vi "Get JSON Data.vi"(6 "Force Hide":bool, 7 "Evaluate Pane Move":bool, 8 "error in (no error)":errorcluster, 9 "Force Get All Data":bool, 10 "VI Reference":refnum<vi>, 11 "String In":refnum<class "String.lvclass">) -> (0 "error out":errorcluster, 2 "JSON string":string, 3 "String Out":refnum<class "String.lvclass">)   [LabVIEW 2017, in "Front Panel Publisher.lvlib" / "String.lvclass"]
uses:
  String.lvclass
  Control_class/Control.lvclass
  Object_class/Object.lvclass
  Web Front Panel_class/Controls/Enum - Control Display Mode.ctl
  Web Front Panel_class/Web Front Panel.lvclass
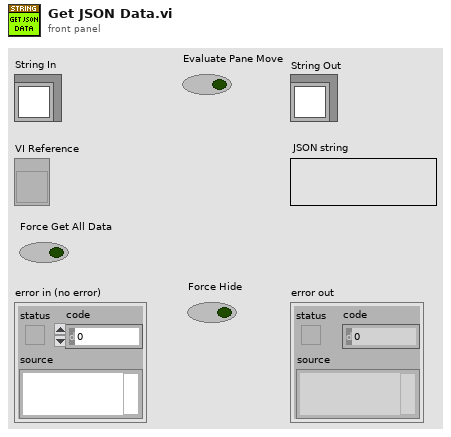
[diagram p1: front panel]
types:
  T1 = typedef "Front Panel Publisher.lvlib/Web Front Panel.lvclass/Enum - Control Display Mode.ctl" = enum16{"Value Only", "Value and Visibility", "Boolean Value Only", "Boolean Value and Visibility", "Control is Image", "Image and Visibility"}
  T2 = typedef "Front Panel Publisher.lvlib/Object.lvclass/Attributes.ctl" = cluster{"UID":i32, "Type":string, "Starting Location":T3, "Reference":refnum<vi>, "Cluster Component":bool, "Starting Rect Position":cluster{"Left":i16, "Top":i16}, "Owning Pane":refnum<vi>, "Master Total Rect Delta":T4}
  T3 = typedef "Front Panel Publisher.lvlib/Object.lvclass/Coordinates.ctl" = cluster{"Left":i32, "Top":i32, "Height":u32, "Width":u32}
  T4 = typedef "LVRectTypeDef.ctl" = cluster{"Left":i16, "Top":i16, "Right":i16, "Bottom":i16}
  T5 = typedef "Front Panel Publisher.lvlib/Control.lvclass/Attributes.ctl" = cluster{"Description":string, "Indicator":bool, "Default Value":variant, "Control Index":i32, "Label":refnum<class "Text.lvclass">, "Caption":refnum<class "Text.lvclass">, "Image b64":string, "No Control Index":bool, "Display Mode":T1}
  T6 = typedef "Front Panel Publisher.lvlib/String.lvclass/Attributes.ctl" = cluster{"String Is Path":bool}
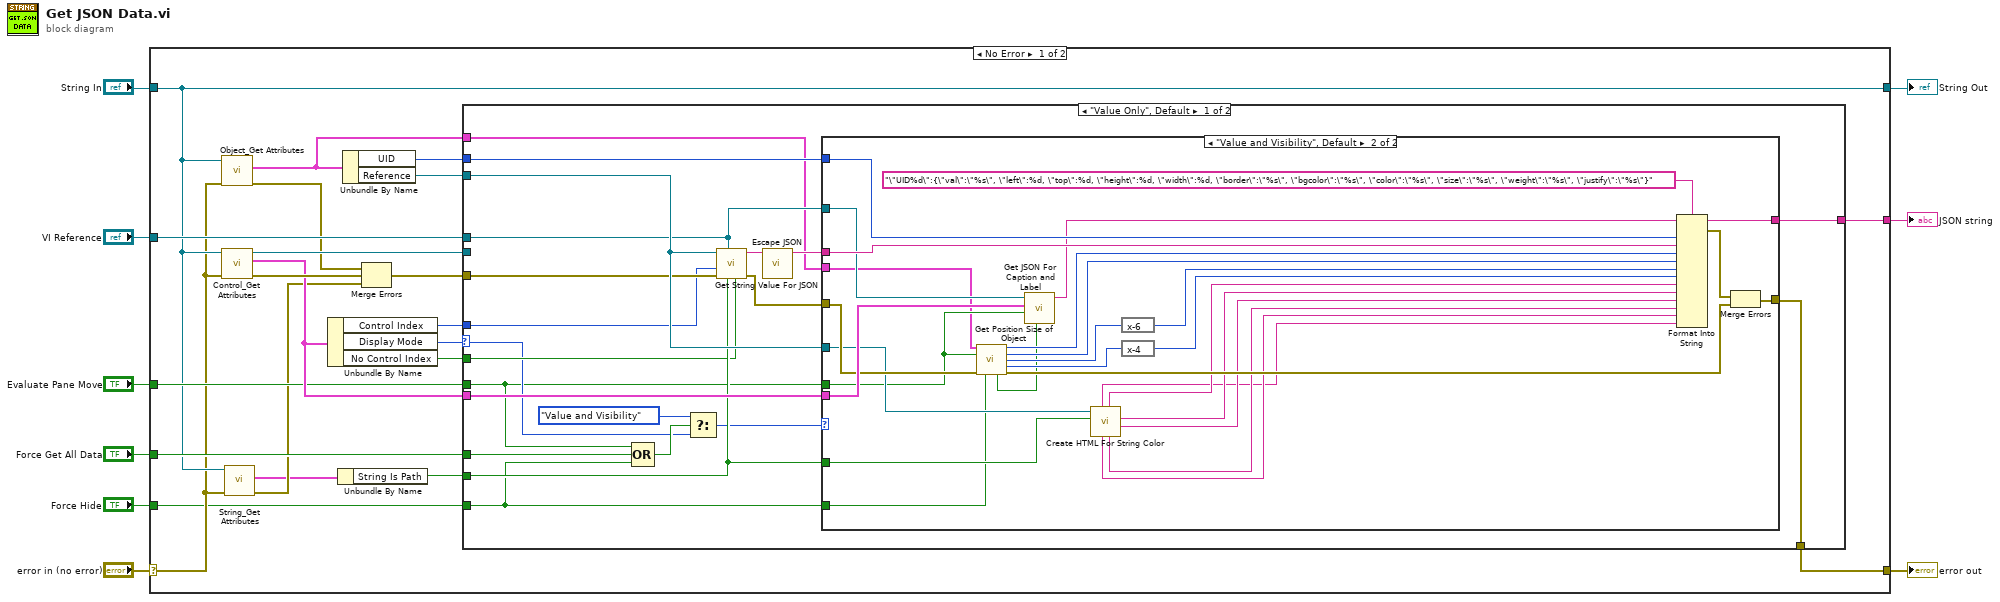
[diagram p0: block diagram]
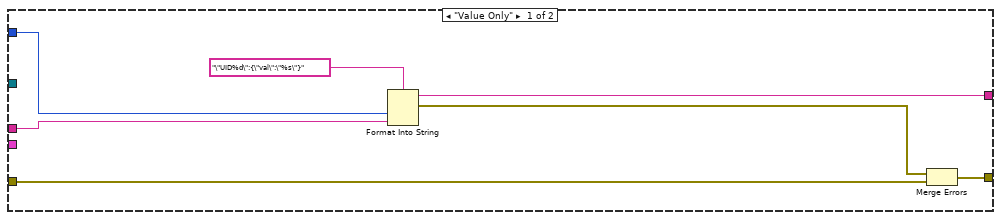
[diagram p2: hidden frame]
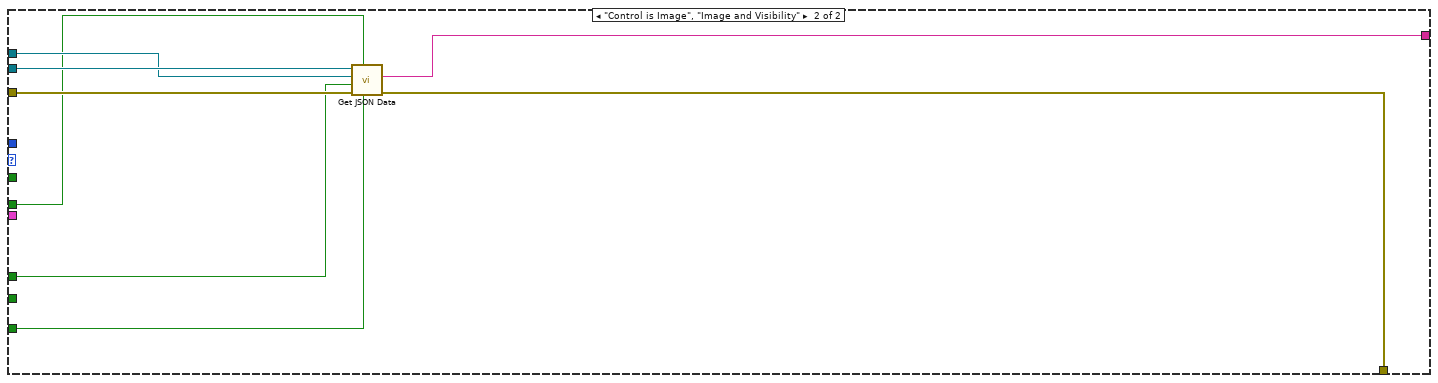
[diagram p3: hidden frame]
diagram:
  n1 = case shown="No Error" "error in (no error)" {
    selector: "error in (no error)" -> [w16 w98]
    tunnel: [w30 w98] -> w8
    tunnel: [w17 w97] -> w6
    tunnel: "String In" -> [w17 w97]
    tunnel: "VI Reference" -> [w28 _]
    tunnel: [w27 _] -> w4
    tunnel: "Force Get All Data" -> [w19 _]
    tunnel: "Evaluate Pane Move" -> [w18 _]
    tunnel: "Force Hide" -> [w11 _]
    frame No Error {
      n2 = call "Object_Get Attributes.vi"("error in (no error)"=w16, "Object In"=w17) -> ("error out"=w21:errorcluster, "Object Attributes"=w10:T2)  [unwired: 7 in, 1 out]
      n3 = call "Control_Get Attributes.vi"("error in (no error)"=w16, "Control In"=w17) -> ("error out"=w31:errorcluster, "Control Attributes"=w20:T5, "Control Out"=w24:refnum<class "String.lvclass">)  [unwired: 7 in]
      n4 = call "String_Get Attributes.vi"("error in (no error)"=w16, "String In"=w17) -> ("error out"=w15:errorcluster, "String Attributes"=w14:T6)  [unwired: 7 in, 1 out]
      n5 = Unbundle By Name(w20) -> ("Control Index"=w29:i32, "Display Mode"=w25:T1, "No Control Index"=w12:bool)
      n6 = Unbundle By Name(w14) -> ("String Is Path"=w13:bool)
      n7 = Unbundle By Name(w10) -> ("UID"=w26:i32, "Reference"=w23:refnum<vi>)
      n8 = Merge Errors(w21, w31, w15) -> (w22:errorcluster)
      n9 = case shown="\"Value Only\", Default" w25 {
        selector: w25 -> [w35 _]
        tunnel: w22 -> [w46 w94]
        tunnel: [w52 w93] -> w30
        tunnel: w29 -> [w45 _]
        tunnel: w28 -> [w47 w95]
        tunnel: [w51 w92] -> w27
        tunnel: w26 -> [w50 _]
        tunnel: w24 -> [_ w96]
        tunnel: w23 -> [w48 _]
        tunnel: w20 -> [w49 _]
        tunnel: w19 -> [w33 w89]
        tunnel: w18 -> [w32 w91]
        tunnel: w13 -> [w44 _]
        tunnel: w12 -> [w40 _]
        tunnel: w11 -> [w34 w90]
        tunnel: w10 -> [w39 _]
        frame "Value Only", Default {
          n10 = Compound Arithmetic op=OR(w32, w33, w34) -> (w37:bool)
          n11 = Select(t=Enum_-_Control_Display_Mode."Value and Visibility", s=w37, f=w35) -> (s? t:f=w36:T1)
          n12 = call "Get String Value For JSON.vi"("No Control Index"=w40, "String Is Path"=w44, "VI Reference"=w47, "error in (no error)"=w46, "Control Index"=w45, "GObject in"=w48) -> ("error out"=w43:errorcluster, "Text"=w42:string)  [unwired: 4 in]
          n13 = call "Escape JSON.vi"("String in"=w42) -> ("String out"=w41:string)  [unwired: 10 in]
          n14 = case shown="\"Value and Visibility\", Default" w36 {
            tunnel: [w57 w86] -> w51
            tunnel: w50 -> [w56 w85]
            tunnel: w41 -> [w55 w84]
            tunnel: w48 -> [_ w71]
            tunnel: [w54 w81] -> w52
            tunnel: w43 -> [w53 w72]
            tunnel: w49 -> [_ w75]
            tunnel: w47 -> [_ w73]
            tunnel: w32 -> [_ w64]
            tunnel: w44 -> [_ w63]
            tunnel: w34 -> [_ w62]
            tunnel: w39 -> [_ w61]
            frame "Value Only" {
              n15 = Format Into String(format string="\"UID%d\":{\"val\":\"%s\"}", w56, w55) -> (resulting string=w57:string, error out=w59:errorcluster)  [unwired: 2 in]
              n16 = Merge Errors(w59, w53) -> (w54:errorcluster)
            }
            frame "Value and Visibility", Default {
              n17 = call "Get Position Size of Object.vi"("Object Attributes"=w61, "Evaluate Pane Move"=w64, "error in (no error)"=w72, "Force Hide"=w62) -> ("Left"=w83:i32, "Top"=w82:i32, "Height"=w79:u32, "Width"=w78:u32, "Hidden"=w60:bool, "error out"=w80:errorcluster)  [unwired: 6 in]
              n18 = call "Get JSON For Caption and Label.vi"("Force Hide"=w60, "Evaluate Pane Move"=w64, "Data"=w75, "VI in"=w73) -> ("JSON"=w74:string)  [unwired: 6 in, 1 out]
              n19 = call "Create HTML For String Color.vi"("String Is Path"=w63, "GObject in"=w71) -> ("Text Color"=w68:string, "Background Color"=w69:string, "Size"=w67:string, "Border"=w70:string, "Weight"=w66:string, "Justify"=w65:string)  [unwired: 2 in, 2 out]
              n20 = expression code="x-6"(w79) -> (w76:u32)
              n21 = expression code="x-4"(w78) -> (w77:u32)
              n22 = Format Into String(format string="\"UID%d\":{\"val\":\"%s\", \"left\":%d, \"top\":%d, \"height\":%d, \"width\":%d, \"border\":\"%s\", \"bgcolor\":\"%s\", \"color\":\"%s\", \"size\":\"%s\", \"weight\":\"%s\", \"justify\":\"%s\"}", initial string=w74, w85, w84, w83, w82, w76, w77, w70, w69, w68, w67, w66, w65) -> (resulting string=w86:string, error out=w88:errorcluster)  [unwired: 1 in]
              n23 = Merge Errors(w88, w80) -> (w81:errorcluster)
            }
          }
        }
        frame "Control is Image", "Image and Visibility" {
          n24 = call-parent "Get JSON Data.vi"("Force Hide"=w90, "Evaluate Pane Move"=w91, "error in (no error)"=w94, "Force Get All Data"=w89, "VI Reference"=w95, "Control In"=w96) -> ("error out"=w93:errorcluster, "JSON string"=w92:string)  [unwired: 3 in, 1 out]
        }
      }
    }
    frame Error {
    }
  }
  "error out" <- w8
  "String Out" <- w6
  "JSON string" <- w4
